vi "random direction.vi"(10 "Directions to Choose From":T1[](array[typedef])) -> (2 "Direction":T1)   [LabVIEW 2015, in "JFD_Common.lvlib"]
uses:
  JFD_Common.lvlib
  Type Defs/Direction Enum.ctl
  Type Defs/SB Type Defs.lvlib
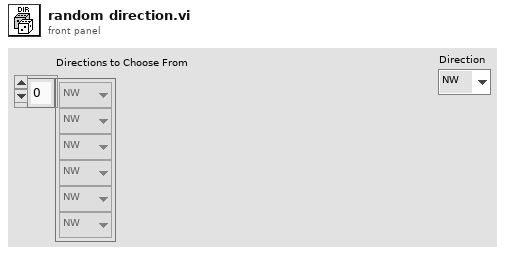
[diagram p1: front panel]
types:
  T1 = typedef "SB Type Defs.lvlib/Direction Enum.ctl" = enum16{"NW", "N", "NE", "E", "SE", "S", "SW", "W"}
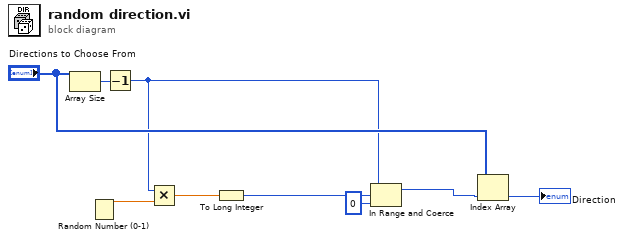
[diagram p0: block diagram]
diagram:
  n1 = Array Size(array="Directions to Choose From") -> (size(s)=w5:i32)
  n2 = Random Number (0-1)() -> (number: 0 to 1=w9:dbl)
  n3 = Decrement(x=w5) -> (x-1=w4:i32)
  n4 = Multiply(x=w4, y=w9) -> (x*y=w8:dbl)
  n5 = To Long Integer(number=w8) -> (32bit integer=w3:i32)
  n6 = In Range and Coerce(upper limit=w4, x=w3, lower limit=0) -> (coerced(x)=w1:i32)  [unwired: 1 out]
  n7 = Index Array(array="Directions to Choose From", index=w1) -> (element=→"Direction":T1)
